vi "Process.vi"(8 "error in":errorcluster, 11 "JKI.Robot.SMO.TestUI":refnum<class "JKI.Robot.SMO.APITesterUI.lvclass">) -> (0 "error out":errorcluster, 3 "JKI.Robot.SMO.TestUI out":refnum<class "JKI.Robot.SMO.APITesterUI.lvclass">)   [LabVIEW 2015, in "JKI.Robot.SMO.APITesterUI.lvclass"]
doc: "---------------------------------------------------------------\nJKI State Machine Objects™\nhttp://jki.net/state-machine-objects/\nCopyright (C) 2005-2015, JKI <info@jki.net>\nALL RIGHTS RESERVEDJKI State Machine Objects (SMO) 1.0.0.5\nJKI - JKI\nCopyright (c) 2016, JKI"
uses:
  JKI.Robot.SMO.APITesterUI.lvclass
  <vilib>/JKI/JKI SMO/SMO/Typedefs/Parent Call--Enum.ctl
  JKI.Robot.SMO.APITesterUI.lvclass/JKI.Robot.SMO.APITesterUI.ctl
  JKI.Robot.SMO.Base/JKI.Robot.SMO.Base.lvclass
  <vilib>/JKI/JKI SMO/SMO.UI/SMO.UI.lvclass
  <vilib>/JKI/JKI SMO/SMO/SMO.lvclass
panel:
  in  "Joint C - Wrist":dbl(knob)=5.611498737356196 scale format="%#.1f"
  in  "Joint B - Elbow":dbl(knob)=5.611498737356196 scale format="%#.1f"
  in  "Joint A - Shoulder":dbl(knob)=5.611498737356196 scale format="%#.1f"
  in  "Claw Value":dbl(slide) scale=0.0..1.0
  # "For instructions on how to use the JKI State Machine Objects, examples and video tutorials, visit:\nhttp://jki.net/state-machine-objects/\n\nJKI State Machine Objects™\nhttp://jki.net/state-machine-objects/\nCopyright (C) 2005-2015, JKI <info@jki.net>\nALL RIGHTS RESERVED"
  # "LABVIEW CONTROLLER"
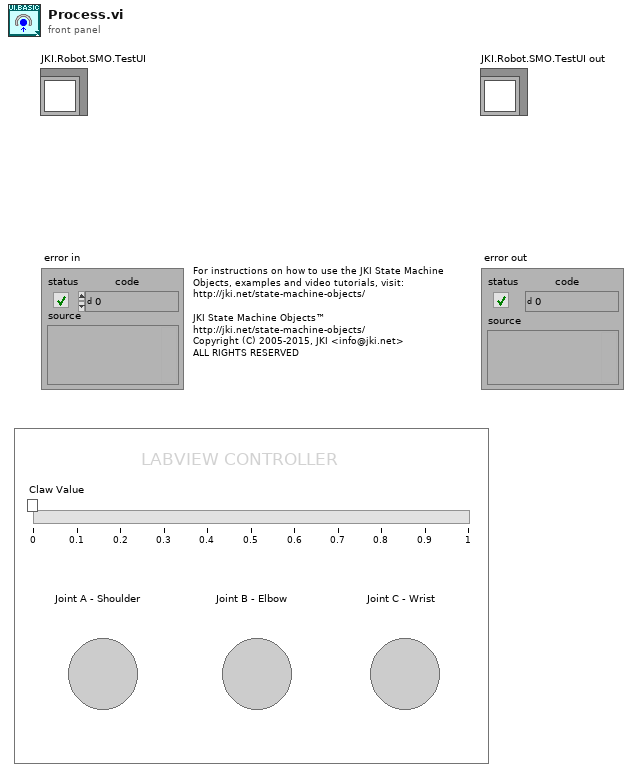
[diagram p1: front panel]
types:
  T1 = typedef "SMO.lvclass/Parent Call--Enum.ctl" = enum16{"Allows parent to run", "Does not request parent to run"}
  T2 = enum32{"invalid app kind", "Development System", "Run Time System", "Student Edition", "Embedded LabVIEW", "Evaluation", "Custom"}
  T3 = enum32{"Invalid", "Standard", "Closed", "Hidden", "Minimized", "Maximized"}
  T4 = cluster{"Core":cluster{"Current VI Reference":refnum<vi>, "Close Panel on Exit?":bool, "error":errorcluster}, "Self Reference":refnum<class "JKI.Robot.SMO.APITesterUI.lvclass">, "JKI.Robot":refnum<class "JKI.Robot.SMO.Base.lvclass">}
  T5 = cluster{"Current VI Reference":refnum<vi>, "Close Panel on Exit?":bool, "error":errorcluster}
  T6 = typedef "SMO.lvclass/Protected Events.ctl" = cluster{"StopProcesses":refnum<user-event>, "AbortProcesses":refnum<user-event>, "Config Changed":refnum<user-event>}
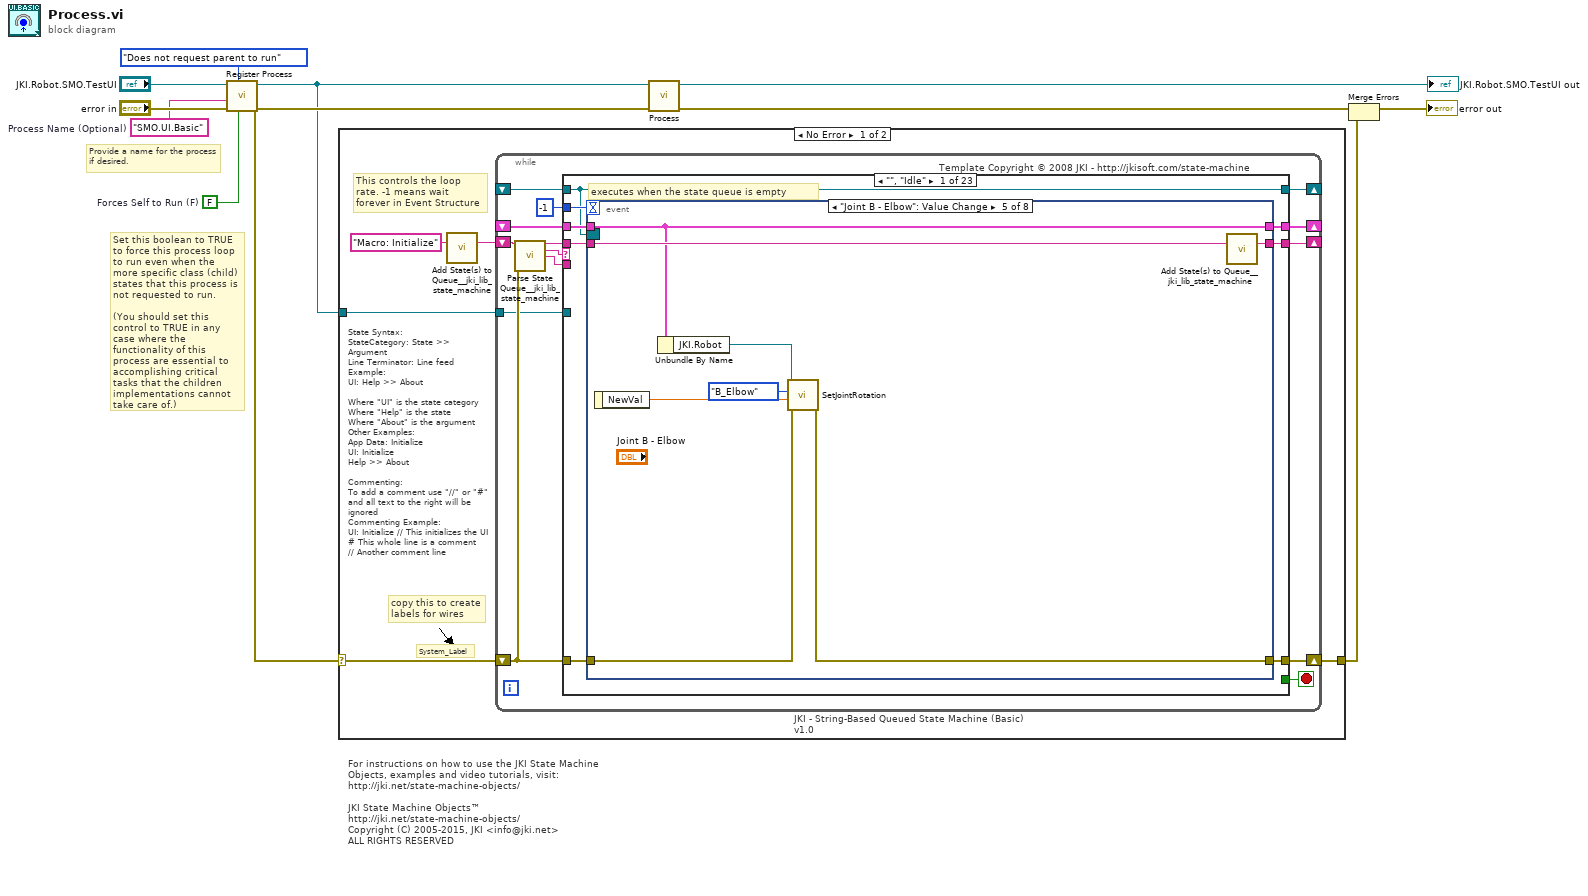
[diagram p0: block diagram]
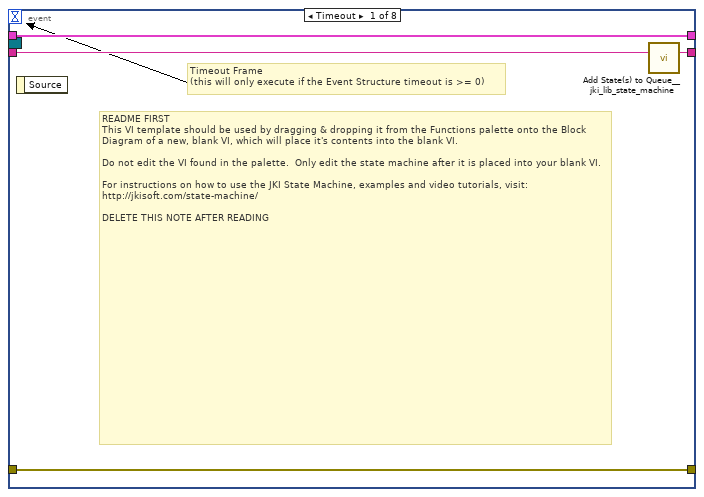
[diagram p2: hidden frame]
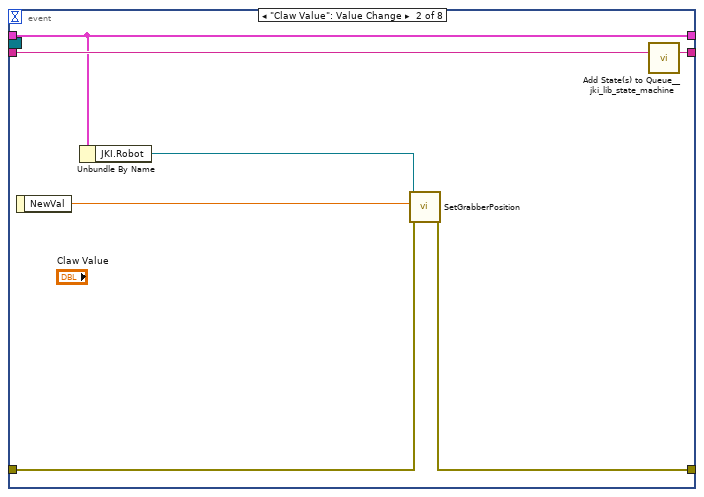
[diagram p3: hidden frame]
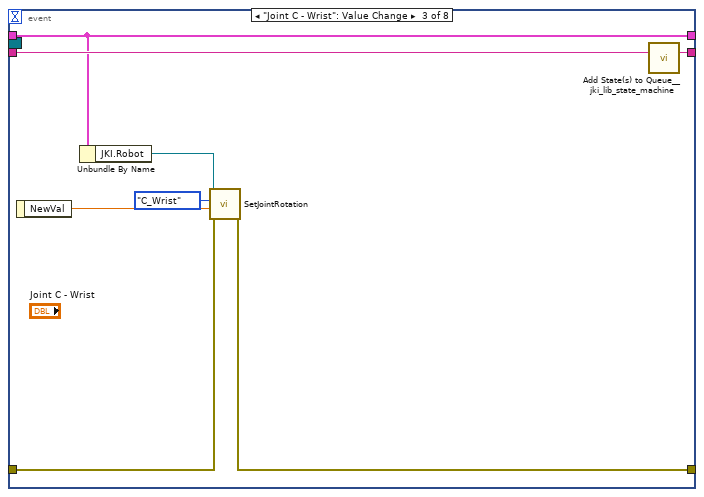
[diagram p4: hidden frame]
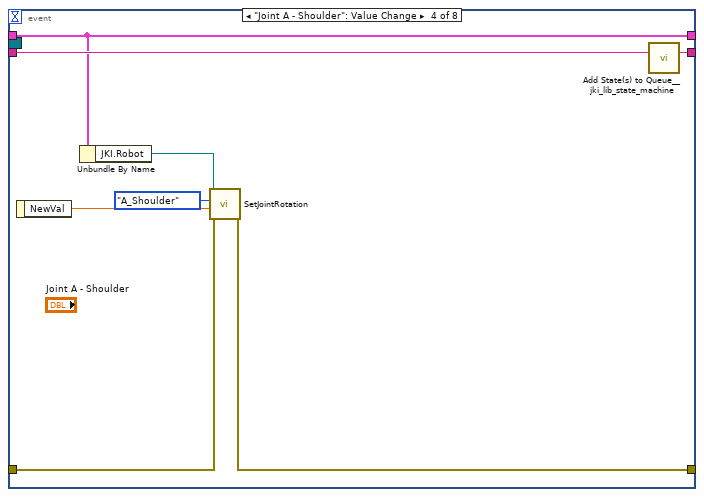
[diagram p5: hidden frame]
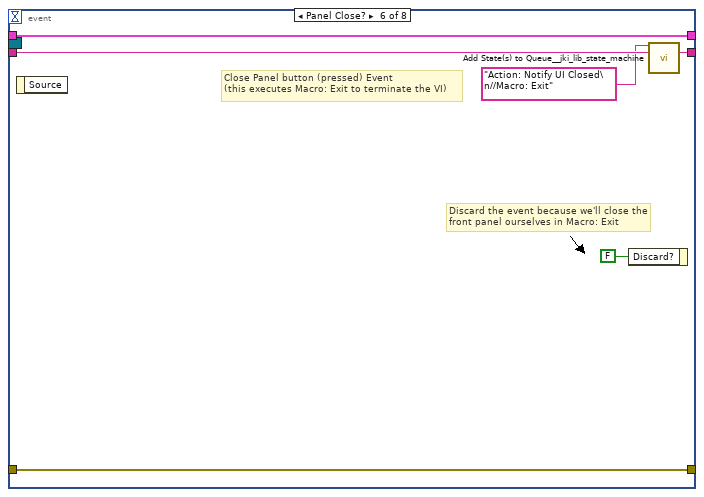
[diagram p6: hidden frame]
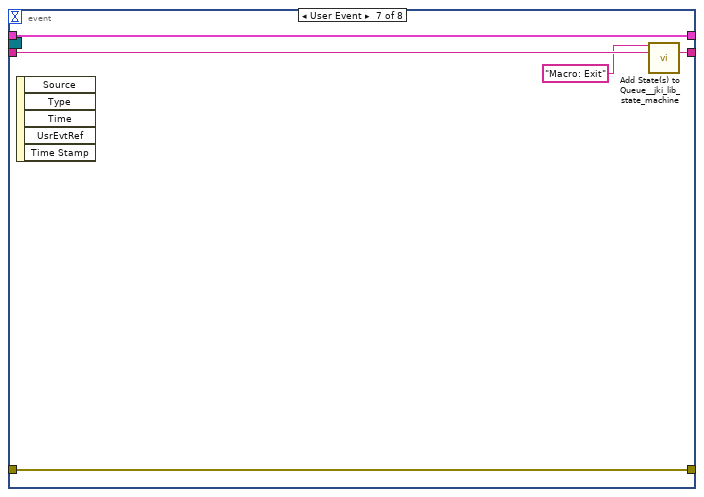
[diagram p7: hidden frame]
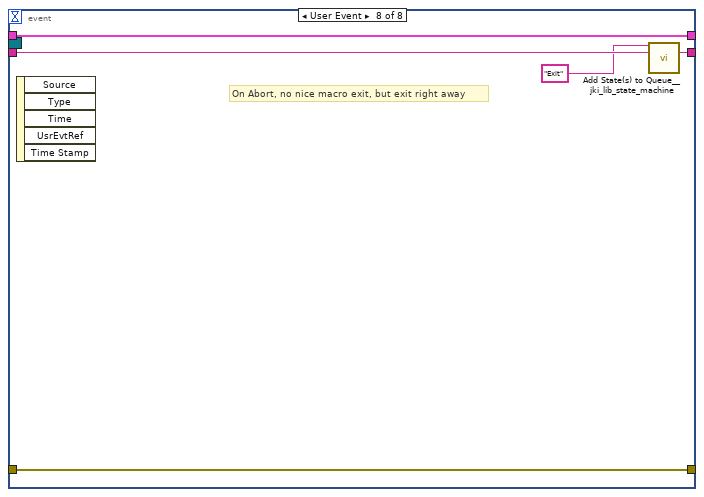
[diagram p8: hidden frame]
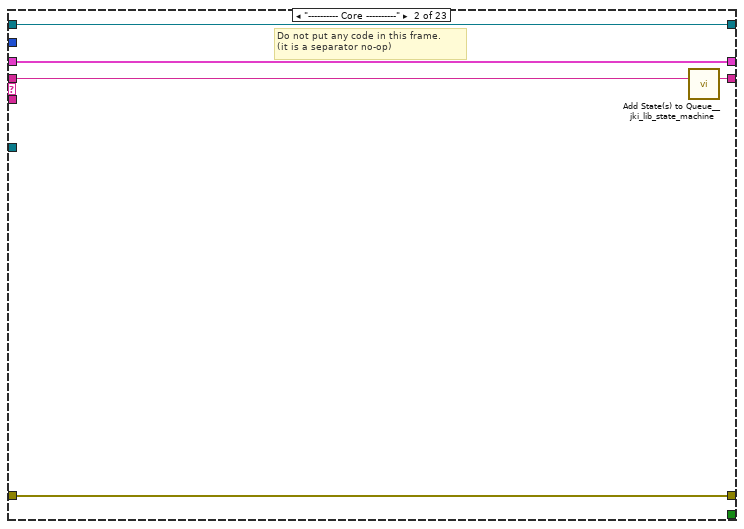
[diagram p9: hidden frame]
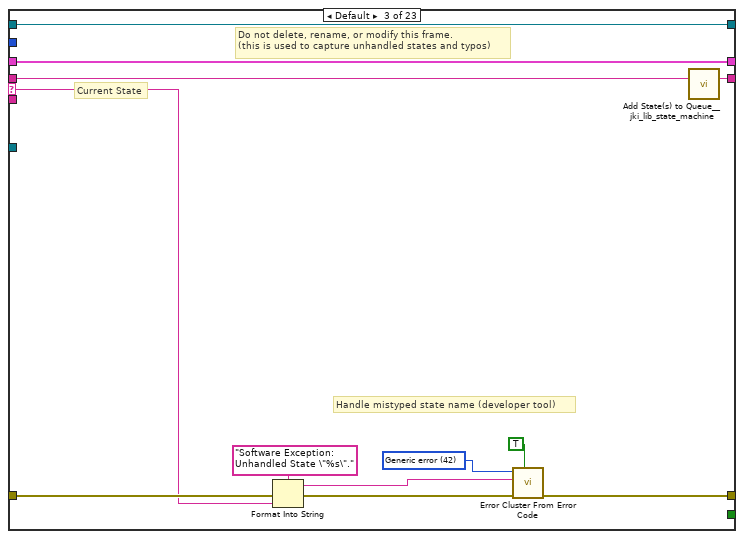
[diagram p10: hidden frame]
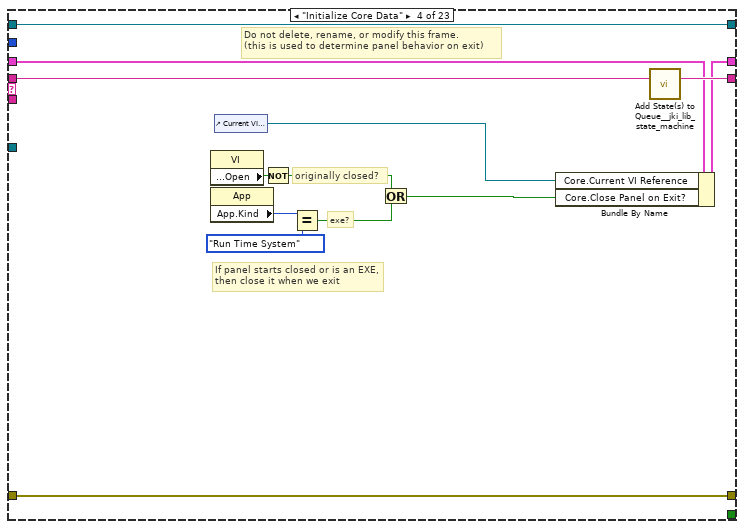
[diagram p11: hidden frame]
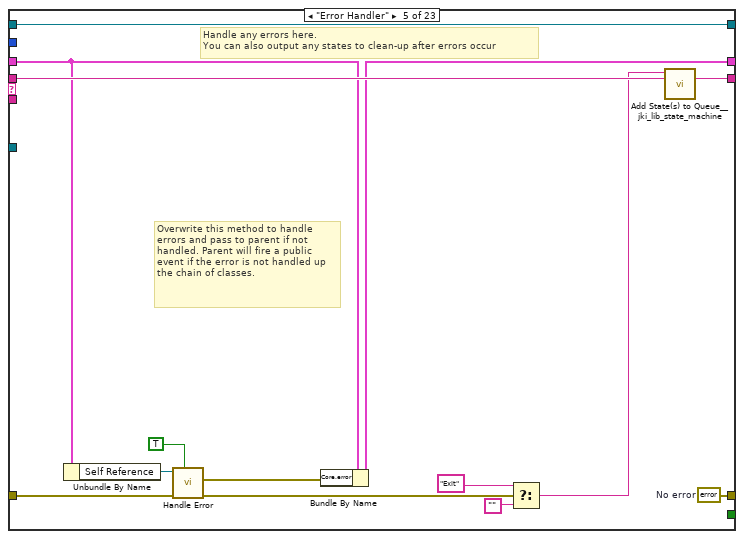
[diagram p12: hidden frame]
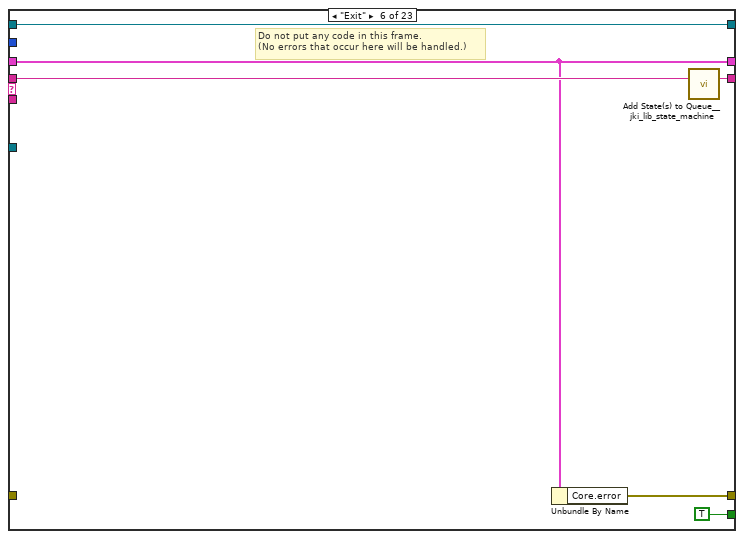
[diagram p13: hidden frame]
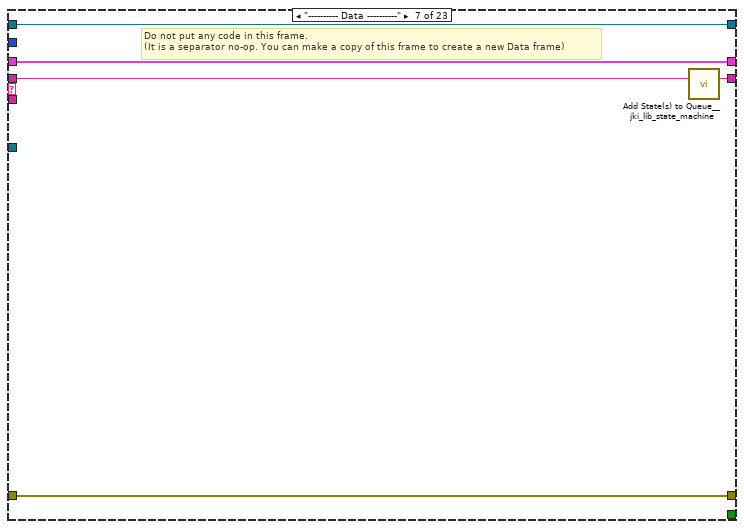
[diagram p14: hidden frame]
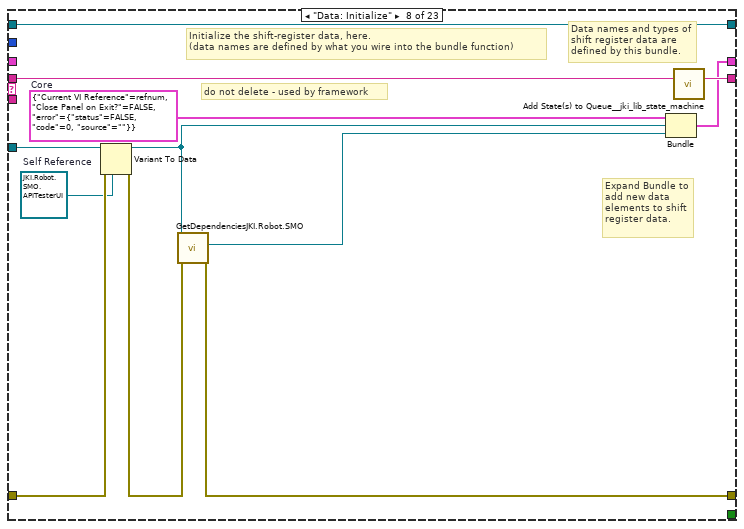
[diagram p15: hidden frame]
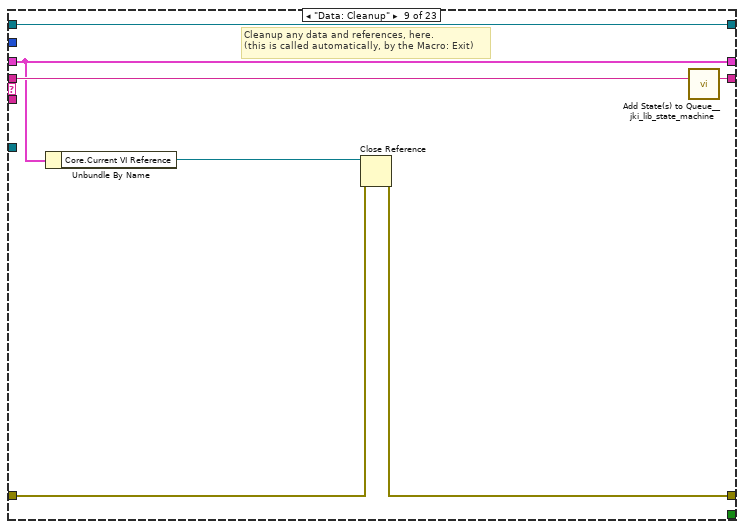
[diagram p16: hidden frame]
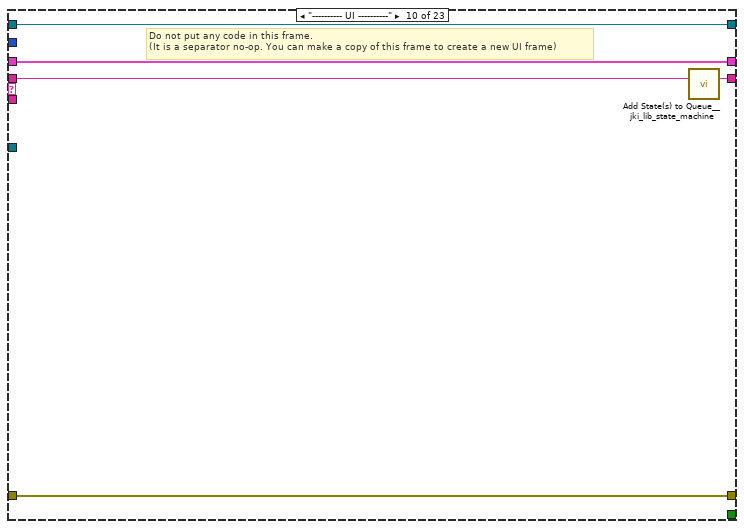
[diagram p17: hidden frame]
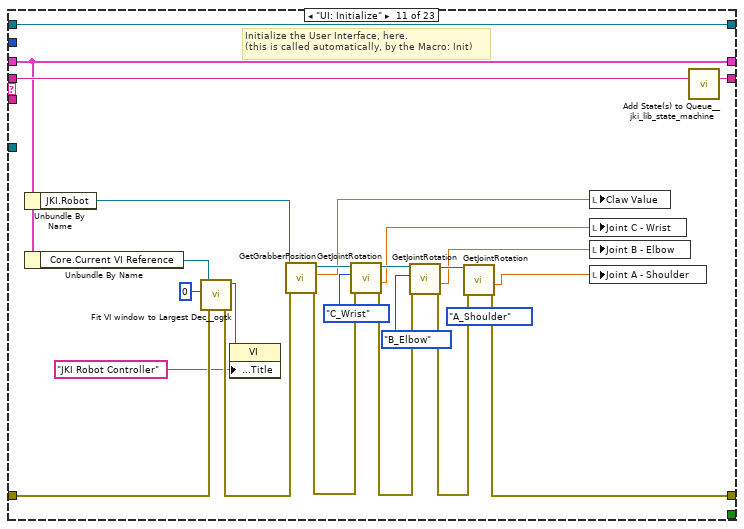
[diagram p18: hidden frame]
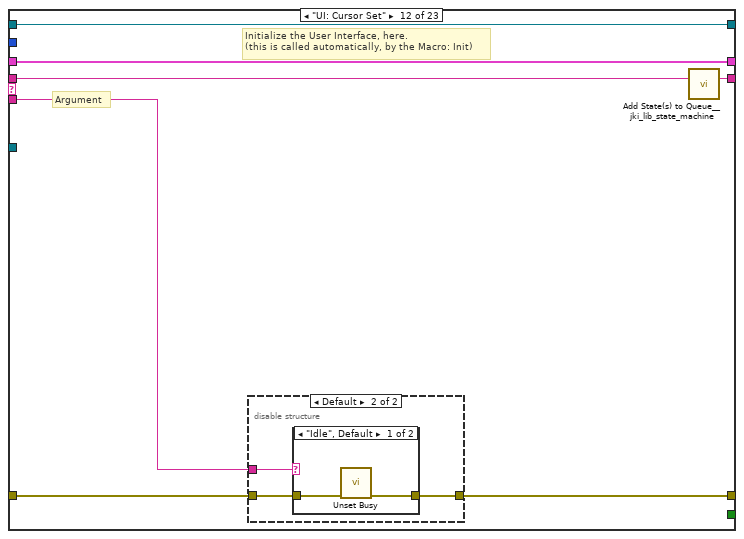
[diagram p19: hidden frame]
diagram:
  w2 = FALSE  # Forces Self to Run (F)
  w1 = "SMO.UI.Basic"  # Process Name (Optional)
  # "Provide a name for the process\nif desired."
  # "Set this boolean to TRUE to force this process loop to run even when the more specific class (child) states that this process is not requested to run.\n\n(You should set this control to TRUE in any case where the functionality of this process are essential to accomplishing critical tasks that the children implementations cannot take care of.)"
  # "For instructions on how to use the JKI State Machine Objects, examples and video tutorials, visit:\nhttp://jki.net/state-machine-objects/\n\nJKI State Machine Objects™\nhttp://jki.net/state-machine-objects/\nCopyright (C) 2005-2015, JKI <info@jki.net>\nALL RIGHTS RESERVED"
  n1 = call <vilib>:"Register Process.vi"("Forces Self to Run (F)"=w2, "Parent Call"=Parent_Call--Enum."Does not request parent to run", "error in (no error)"="error in", "Process Name (optional)"=w1, "SMO"="JKI.Robot.SMO.TestUI") -> ("error out"=w8:errorcluster, "SMO out"=w7:refnum<class "JKI.Robot.SMO.APITesterUI.lvclass">)  [unwired: 5 in]
  n2 = case shown="No Error" w8 {
    selector: w8 -> [w13 w333]
    tunnel: w7 -> [w14 _]
    tunnel: [w12 w333] -> w4
    frame No Error {
      # "State Syntax:\nStateCategory: State >> Argument\nLine Terminator: Line feed\nExample:\nUI: Help >> About\n\nWhere \"UI\" is the state category\nWhere \"Help\" is the state\nWhere \"About\" is the argument\nOther Examples:\nApp Data: Initialize\nUI: Initialize\nHelp >> About\n\nCommenting:\nTo add a comment use \"//\" or \"#\" and all text to the right will be ignored\nCommenting Example:\nUI: Initialize // This initializes the UI\n# This whole line is a comment\n// Another comment line"
      # "copy this to create labels for wires"
      # "This controls the loop rate. -1 means wait forever in Event Structure"
      # "System_Label"
      n3 = call <vilib>:"Add State(s) to Queue__jki_lib_state_machine.vi"("State(s) in (\"\")"="Macro: Initialize") -> ("States Out"=w16:string)  [unwired: 14 in]
      n4 = while "JKI - String-Based Queued State Machine (Basic) v1.0" {
        shift-right: [w23] -> _
        shift-left: _ -> [w22]
        shift-right: [w26] -> w12
        shift-left: w13 -> [w20]
        shift-right: [w25] -> _
        shift-left: w16 -> [w27]
        tunnel: w14 -> [w19]
        shift-right: [w18] -> _
        shift-left: _ -> [w17]
        stop <- w24 stop-if-true
        # "Template Copyright © 2008 JKI - http://jkisoft.com/state-machine"
        n5 = call <vilib>:"Parse State Queue__jki_lib_state_machine.vi"("State Queue"=w27, "Error In (no error)"=w20) -> ("Remaining States"=w29:string, "Current State"=w30:string, "Arguments"=w28:string)  [unwired: 11 in]
        n6 = case shown="\"\", \"Idle\"" w30 {
          selector: w30 -> [_ _ w96 _ _ _ _ _ _ _ _ _ _ _ _ _ _ _ _ _ _ _ _]
          tunnel: w29 -> [w38 w94 w100 w119 w133 w139 w144 w156 w163 w168 w193 w200 w216 w248 w257 w271 w276 w287 w292 w303 w318 w325 w332]
          tunnel: w28 -> [_ _ _ _ _ _ _ _ _ _ _ w194 w210 _ _ _ _ _ _ _ _ _ _]
          tunnel: w22 -> [w36 w91 w98 w110 w122 w135 w141 _ w158 w165 w174 w198 w212 w245 w253 w262 w273 w284 w289 w301 w316 w321 w328]
          tunnel: [w35 w92 w102 w116 w124 w134 w142 w146 w159 w166 w183 w195 w213 w246 w255 w269 w274 w278 w290 w299 w313 w322 w326] -> w26
          tunnel: w20 -> [w34 w92 w101 w116 w129 _ w142 w153 w160 w166 w172 w196 w214 w246 w255 w269 w274 w279 w290 w300 w314 w322 w327]
          tunnel: [w37 w93 w99 w118 w132 w138 w143 w155 w162 w167 w192 w199 w215 w247 w256 w270 w275 w286 w291 w302 w317 w324 w331] -> w25
          tunnel: [_ _ _ _ _ TRUE _ _ _ _ _ _ _ _ _ _ _ _ _ _ _ _ _] -> w24
          tunnel: [w33 w91 w98 w117 w121 w135 w141 w154 w158 w165 w174 w198 w212 w245 w253 w262 w273 w284 w289 w301 w316 w320 w328] -> w23
          tunnel: -1 ("Timeout") -> [w32 _ _ _ _ _ _ _ _ _ _ _ _ _ _ _ _ _ _ _ _ _ _]
          tunnel: w19 -> [_ _ _ _ _ _ _ w151 _ _ _ _ _ _ _ _ _ _ _ _ _ _ _]
          tunnel: [w31 w90 w95 w107 w131 w136 w140 w150 w157 w164 w191 w197 w209 w244 w254 w263 w272 w285 w288 w298 w315 w323 w330] -> w18
          tunnel: w17 -> [w31 w90 w95 w107 w131 w136 w140 w150 w157 w164 w191 w197 w209 w244 w254 w263 w272 w285 w288 w294 w315 w323 w330]
          frame "", "Idle" {
            # "executes when the state queue is empty"
            n7 = event shown="[4] \"Joint B - Elbow\": Value Change" {
              selector: w31 -> [_ _ _ _ _ _ _ _]
              dyn-events: _ -> [_ _ _ _ _ _ _ _]
              timeout: w32 -> [_ _ _ _ _ _ _ _]
              tunnel: w38 -> [w42 w49 w57 w65 w73 w79 w84 w89]
              tunnel: [w41 w48 w56 w64 w72 w78 w83 w88] -> w37
              tunnel: w36 -> [w39 w47 w55 w63 w71 w75 w81 w86]
              tunnel: [w40 w43 w52 w60 w68 w74 w82 w87] -> w35
              tunnel: w34 -> [w40 w44 w53 w61 w69 w74 w82 w87]
              tunnel: [w39 w47 w55 w63 w71 w75 w81 w86] -> w33
              event Timeout {
                # "README FIRST\nThis VI template should be used by dragging & dropping it from the Functions palette onto the Block Diagram of a new, blank VI, which will place it's contents into the blank VI.\n\nDo not edit the VI found in the palette.  Only edit the state machine after it is placed into your blank VI.\n\nFor instructions on how to use the JKI State Machine, examples and video tutorials, visit:\nhttp://jkisoft.com/state-machine/\n\nDELETE THIS NOTE AFTER READING"
                # "Timeout Frame\n(this will only execute if the Event Structure timeout is >= 0)"
                n8 = event-data() -> ()  [unwired: 1 in, 1 out]
                n9 = call <vilib>:"Add State(s) to Queue__jki_lib_state_machine.vi"("State(s) in (\"\")"=w42) -> ("States Out"=w41:string)  [unwired: 14 in]
              }
              event "Claw Value": Value Change {
                n10 = event-data() -> ("NewVal"=w45:dbl)  [unwired: 1 in]
                n11 = Unbundle By Name(w47) -> ("JKI.Robot"=w46:refnum<class "JKI.Robot.SMO.Base.lvclass">)
                n12 = call-dynamic "SetGrabberPosition.vi"("error in (no error)"=w44, "GrabberPosition"=w45, "JKI.Robot"=w46) -> ("error out"=w43:errorcluster)  [unwired: 7 in, 1 out]
                n13 = call <vilib>:"Add State(s) to Queue__jki_lib_state_machine.vi"("State(s) in (\"\")"=w49) -> ("States Out"=w48:string)  [unwired: 14 in]
              }
              event "Joint C - Wrist": Value Change {
                n14 = event-data() -> ("NewVal"=w51:dbl)  [unwired: 1 in]
                n15 = Unbundle By Name(w55) -> ("JKI.Robot"=w54:refnum<class "JKI.Robot.SMO.Base.lvclass">)
                n16 = call-dynamic "SetJointRotation.vi"("error in (no error)"=w53, "Rotation (Deg)"=w51, "Joint"=enum16{"A_Shoulder", "B_Elbow", "C_Wrist"}."C_Wrist" ("JointType"), "JKI.Robot.SMO.Base"=w54) -> ("error out"=w52:errorcluster)  [unwired: 6 in, 1 out]
                n17 = call <vilib>:"Add State(s) to Queue__jki_lib_state_machine.vi"("State(s) in (\"\")"=w57) -> ("States Out"=w56:string)  [unwired: 14 in]
              }
              event "Joint A - Shoulder": Value Change {
                n18 = event-data() -> ("NewVal"=w59:dbl)  [unwired: 1 in]
                n19 = Unbundle By Name(w63) -> ("JKI.Robot"=w62:refnum<class "JKI.Robot.SMO.Base.lvclass">)
                n20 = call-dynamic "SetJointRotation.vi"("error in (no error)"=w61, "Rotation (Deg)"=w59, "Joint"=enum16{"A_Shoulder", "B_Elbow", "C_Wrist"}."A_Shoulder" ("JointType"), "JKI.Robot.SMO.Base"=w62) -> ("error out"=w60:errorcluster)  [unwired: 6 in, 1 out]
                n21 = call <vilib>:"Add State(s) to Queue__jki_lib_state_machine.vi"("State(s) in (\"\")"=w65) -> ("States Out"=w64:string)  [unwired: 14 in]
              }
              event "Joint B - Elbow": Value Change {
                n22 = event-data() -> ("NewVal"=w67:dbl)  [unwired: 1 in]
                n23 = Unbundle By Name(w71) -> ("JKI.Robot"=w70:refnum<class "JKI.Robot.SMO.Base.lvclass">)
                n24 = call-dynamic "SetJointRotation.vi"("error in (no error)"=w69, "Rotation (Deg)"=w67, "Joint"=enum16{"A_Shoulder", "B_Elbow", "C_Wrist"}."B_Elbow" ("JointType"), "JKI.Robot.SMO.Base"=w70) -> ("error out"=w68:errorcluster)  [unwired: 6 in, 1 out]
                n25 = call <vilib>:"Add State(s) to Queue__jki_lib_state_machine.vi"("State(s) in (\"\")"=w73) -> ("States Out"=w72:string)  [unwired: 14 in]
              }
              event Panel Close? {
                # "Discard the event because we'll close the front panel ourselves in Macro: Exit"
                # "Close Panel button (pressed) Event\n(this executes Macro: Exit to terminate the VI)"
                n26 = event-data() -> ()  [unwired: 1 in, 1 out]
                n27 = event-data("Discard?"=FALSE) -> ()  [unwired: 1 in, 1 out]
                n28 = call <vilib>:"Add State(s) to Queue__jki_lib_state_machine.vi"("State(s) in Front (\"\")"="Action: Notify UI Closed\n//Macro: Exit", "State(s) in (\"\")"=w79) -> ("States Out"=w78:string)  [unwired: 13 in]
              }
              event User Event {
                n29 = event-data() -> ()  [unwired: 1 in, 5 out]
                n30 = call <vilib>:"Add State(s) to Queue__jki_lib_state_machine.vi"("State(s) in Front (\"\")"="Macro: Exit", "State(s) in (\"\")"=w84) -> ("States Out"=w83:string)  [unwired: 13 in]
              }
              event User Event {
                # "On Abort, no nice macro exit, but exit right away"
                n31 = event-data() -> ()  [unwired: 1 in, 5 out]
                n32 = call <vilib>:"Add State(s) to Queue__jki_lib_state_machine.vi"("State(s) in Front (\"\")"="Exit", "State(s) in (\"\")"=w89) -> ("States Out"=w88:string)  [unwired: 13 in]
              }
            }
          }
          frame "---------- Core ----------" {
            # "Do not put any code in this frame.\n(it is a separator no-op)"
            n33 = call <vilib>:"Add State(s) to Queue__jki_lib_state_machine.vi"("State(s) in (\"\")"=w94) -> ("States Out"=w93:string)  [unwired: 14 in]
          }
          frame Default {
            w105 = 42 items=["No error", "Argument error", "Memory is full", "Out of zone", "End of file", "File already open", "Generic file I/O error", "File not found", "File permission error", "Disk is full", "Duplicate path", "Too many files open", "System feature not enabled", "Resource file not found", "Cannot add resource", "Resource not found", "Image not found", "Image memory error", "Pen does not exist", "Config type invalid", "Config token not found", "Config parse error", "Config memory error", "Bad external code format", "Bad external code offset", "External code not present", "Null window", "Destroy window error", "Null menu", "Print aborted", "Bad print record", "Print driver error", "Windows error during printing", "Memory error during printing", "Print dialog error", "Generic print error", "Invalid device refnum", "Device not found", "Device parameter error", "Device unit error", "Cannot open device", "Device call aborted", "Generic error", "Cancelled by user", "Object ID too low", "Object ID too high", "Object not in heap", "Unknown heap", "Unknown object (invalid DefProc)", "Unknown object (DefProc not in table)", "Message out of range", "Invalid (null) method", "Unknown message", "Manager call not supported", "Bad address", "Network operation in progress", "Network operation timed out", "Connection is busy", "Network attribute not supported", "Network error", "Address in use", "System out of memory", "Connection aborted", "Connection refused", "Not connected", "Already connected", "Connection closed", "Initialization error (interapplication manager)", "Bad occurrence", "Wait on unbound occurrence handler", "Occurrence queue overflow", "Datalog type conflict", "Unused", "Unrecognized type (interapplication manager)", "Memory corrupt", "Failed to make temporary DLL", "Old CIN version", "Drag socket not found", "Failed to load drop-object", "Failed to register OLE object", "Failed to release OLE object", "Format specifier type mismatch", "Unknown format specifier", "Too few format specifiers", "Too many format specifiers", "Scan failed", "Newer CIN version", "Error converting to variant", "Runtime menu error", "Password tampered", "Variant attribute not found", "Incompatible variant data type", "Event data is not available", "Event Store is not present", "Occurrence is not found", "Event Queue is not created", "Event info is not available", "Refnum passed is NULL", "Error retrieving Class GUID", "Error retrieving CoClass GUID", "Error retrieving TypeLib GUID.", "Bad built application magic bytes.", "Specific driver is different from the specific driver associated with the Logical Name.", "There is no session opened to the class driver.", "Max Error", "MAX - Error with config objects", "MAX - Error loading configuration", "MAX - Group not supported"]
            # "Current State"
            # "Do not delete, rename, or modify this frame.\n(this is used to capture unhandled states and typos)"
            # "Handle mistyped state name (developer tool)"
            n34 = Format Into String(format string="Software Exception: Unhandled State \"%s\"." ("message"), error in=w101, w96) -> (resulting string=w104:string, error out=w103:errorcluster)  [unwired: 1 in]
            n35 = call <vilib>:"Error Cluster From Error Code.vi"("show call chain? (False)"=TRUE, "error in (no error)"=w103, "error message (\"\")"=w104, "error code (0)"=w105) -> ("error out"=w102:errorcluster)  [unwired: 5 in]
            n36 = call <vilib>:"Add State(s) to Queue__jki_lib_state_machine.vi"("State(s) in (\"\")"=w100) -> ("States Out"=w99:string)  [unwired: 14 in]
          }
          frame "Initialize Core Data" {
            # "Do not delete, rename, or modify this frame.\n(this is used to determine panel behavior on exit)"
            # "originally closed?"
            # "exe?"
            # "If panel starts closed or is an EXE, then close it when we exit"
            n37 = property class="VI"() -> ("Front Panel.Open"=w115:bool)  [unwired: 2 in, 2 out]
            n38 = property class="App"() -> ("App.Kind"=w114:T2)  [unwired: 2 in, 2 out]
            n39 = control-ref of="Current VI Reference"() -> (w108:refnum<vi>)
            n40 = Not(x=w115) -> (.not. x?=w112:bool)
            n41 = Equal?(x=w114, y=T2."Run Time System" ("Application:Kind")) -> (x = y?=w111:bool)
            n42 = Or(x=w112, y=w111) -> (x .or. y?=w109:bool)
            n43 = Bundle By Name(cluster=w110, "Core.Current VI Reference"=w108, "Core.Close Panel on Exit?"=w109) -> (w117:T4)
            n44 = call <vilib>:"Add State(s) to Queue__jki_lib_state_machine.vi"("State(s) in (\"\")"=w119) -> ("States Out"=w118:string)  [unwired: 14 in]
          }
          frame "Error Handler" {
            w124 = errorcluster {"status"=FALSE, "code"=0, "source"=""}  # No error
            # "Overwrite this method to handle errors and pass to parent if not handled. Parent will fire a public event if the error is not handled up the chain of classes."
            # "Handle any errors here.\nYou can also output any states to clean-up after errors occur"
            n45 = Unbundle By Name(w122) -> ("Self Reference"=w130:refnum<class "JKI.Robot.SMO.APITesterUI.lvclass">)
            n46 = call-dynamic "Handle Error.vi"("Stop on Unhandled Error (T)"=TRUE, "error in"=w129, "SMO"=w130) -> ("handling error"=w125:errorcluster, "Unhandled error"=w123:errorcluster)  [unwired: 6 in, 1 out]
            n47 = Bundle By Name(cluster=w122, "Core.error"=w123) -> (w121:T4)
            n48 = Select(t="Exit", s=w125, f="") -> (s? t:f=w126:string)
            n49 = call <vilib>:"Add State(s) to Queue__jki_lib_state_machine.vi"("State(s) in Front (\"\")"=w126, "State(s) in (\"\")"=w133) -> ("States Out"=w132:string)  [unwired: 13 in]
          }
          frame "Exit" {
            # "Do not put any code in this frame.\n(No errors that occur here will be handled.)"
            n50 = Unbundle By Name(w135) -> ("Core.error"=w134:errorcluster)
            n51 = call <vilib>:"Add State(s) to Queue__jki_lib_state_machine.vi"("State(s) in (\"\")"=w139) -> ("States Out"=w138:string)  [unwired: 14 in]
          }
          frame "---------- Data ----------" {
            # "Do not put any code in this frame.\n(It is a separator no-op. You can make a copy of this frame to create a new Data frame)"
            n52 = call <vilib>:"Add State(s) to Queue__jki_lib_state_machine.vi"("State(s) in (\"\")"=w144) -> ("States Out"=w143:string)  [unwired: 14 in]
          }
          frame "Data: Initialize" {
            w149 = T5 {"Current VI Reference"=refnum, "Close Panel on Exit?"=FALSE, "error"={"status"=FALSE, "code"=0, "source"=""}}  # Core
            w152 = refnum<class "JKI.Robot.SMO.APITesterUI.lvclass"> refnum  # Self Reference
            # "do not delete - used by framework"
            # "Expand Bundle to add new data elements to shift register data."
            # "Data names and types of shift register data are defined by this bundle."
            # "Initialize the shift-register data, here.\n(data names are defined by what you wire into the bundle function)"
            n53 = Variant To Data(error in=w153, type=w152, Variant=w151) -> (data=w148:refnum<class "JKI.Robot.SMO.APITesterUI.lvclass">, error out=w147:errorcluster)
            n54 = call "GetDependenciesJKI.Robot.SMO.vi"("error in (no error)"=w147, "JKI.Robot.SMO.APITesterUI in"=w148) -> ("error out"=w146:errorcluster, "JKI.Robot"=w145:refnum<class "JKI.Robot.SMO.Base.lvclass">)  [unwired: 7 in, 1 out]
            n55 = Bundle("Core"=w149, "Self Reference"=w148, "JKI.Robot"=w145) -> (w154:T4)  [unwired: 1 in]
            n56 = call <vilib>:"Add State(s) to Queue__jki_lib_state_machine.vi"("State(s) in (\"\")"=w156) -> ("States Out"=w155:string)  [unwired: 14 in]
          }
          frame "Data: Cleanup" {
            # "Cleanup any data and references, here.\n(this is called automatically, by the Macro: Exit)"
            n57 = Unbundle By Name(w158) -> ("Core.Current VI Reference"=w161:refnum<vi>)
            n58 = Close Reference(reference=w161, error in (no error)=w160) -> (error out=w159:errorcluster)
            n59 = call <vilib>:"Add State(s) to Queue__jki_lib_state_machine.vi"("State(s) in (\"\")"=w163) -> ("States Out"=w162:string)  [unwired: 14 in]
          }
          frame "---------- UI ----------" {
            # "Do not put any code in this frame.\n(It is a separator no-op. You can make a copy of this frame to create a new UI frame)"
            n60 = call <vilib>:"Add State(s) to Queue__jki_lib_state_machine.vi"("State(s) in (\"\")"=w168) -> ("States Out"=w167:string)  [unwired: 14 in]
          }
          frame "UI: Initialize" {
            # "Initialize the User Interface, here.\n(this is called automatically, by the Macro: Init)"
            n61 = Unbundle By Name(w174) -> ("JKI.Robot"=w190:refnum<class "JKI.Robot.SMO.Base.lvclass">)
            n62 = Unbundle By Name(w174) -> ("Core.Current VI Reference"=w173:refnum<vi>)
            n63 = call <userlib>:"Fit VI window to Largest Dec__ogtk.vi"("error in (no error)"=w172, "border spacing (2 px)"=0, "VI Ref (calling VI)"=w173) -> ("error out"=w171:errorcluster, "dup VI Ref"=w170:refnum<vi>)  [unwired: 3 in]
            n64 = property class="VI"(reference=w170, "Front Panel.Title"="JKI Robot Controller" ("Front Panel Window:Title")) -> ()  [unwired: 1 in, 2 out]
            n65 = call-dynamic "GetGrabberPosition.vi"("error in (no error)"=w171, "JKI.Robot.SMO.Base.lvclass"=w190) -> ("error out"=w186:errorcluster, "SetGrabberPosition"=w182:dbl, "JKI.Robot.SMO.Base.lvclass"=w189:refnum<class "JKI.Robot.SMO.Base.lvclass">)  [unwired: 7 in]
            n66 = call-dynamic "GetJointRotation.vi"("error in (no error)"=w186, "Joint"=enum16{"A_Shoulder", "B_Elbow", "C_Wrist"}."C_Wrist" ("JointType"), "JKI.Robot.SMO.Base"=w189) -> ("error out"=w185:errorcluster, "Rotation (Deg)"=w181:dbl, "JKI.Robot.SMO.Base"=w188:refnum<class "JKI.Robot.SMO.Base.lvclass">)  [unwired: 6 in]
            n67 = call-dynamic "GetJointRotation.vi"("error in (no error)"=w185, "Joint"=enum16{"A_Shoulder", "B_Elbow", "C_Wrist"}."B_Elbow" ("JointType"), "JKI.Robot.SMO.Base"=w188) -> ("error out"=w184:errorcluster, "Rotation (Deg)"=w180:dbl, "JKI.Robot.SMO.Base"=w187:refnum<class "JKI.Robot.SMO.Base.lvclass">)  [unwired: 6 in]
            n68 = call-dynamic "GetJointRotation.vi"("error in (no error)"=w184, "Joint"=enum16{"A_Shoulder", "B_Elbow", "C_Wrist"}."A_Shoulder" ("JointType"), "JKI.Robot.SMO.Base"=w187) -> ("error out"=w183:errorcluster, "Rotation (Deg)"=w179:dbl)  [unwired: 6 in, 1 out]
            n69 = local write "Claw Value"(w182) -> ()
            n70 = local write "Joint C - Wrist"(w181) -> ()
            n71 = local write "Joint B - Elbow"(w180) -> ()
            n72 = local write "Joint A - Shoulder"(w179) -> ()
            n73 = call <vilib>:"Add State(s) to Queue__jki_lib_state_machine.vi"("State(s) in (\"\")"=w193) -> ("States Out"=w192:string)  [unwired: 14 in]
          }
          frame "UI: Cursor Set" {
            # "Argument"
            # "Initialize the User Interface, here.\n(this is called automatically, by the Macro: Init)"
            n74 = disable-structure shown="Default" {
              disable-tunnel: w196 -> [w201 w204]
              disable-tunnel: [w201 w203] -> w195
              disable-tunnel: w194 -> [_ w202]
              frame condition #0 {
              }
              frame condition #1 (active) {
                n75 = case shown="\"Idle\", Default" w202 {
                  tunnel: w204 -> [w206 w208]
                  tunnel: [w205 w207] -> w203
                  frame "Idle", Default {
                    n76 = call <vilib>:"Unset Busy.vi"("error in (no error)"=w206) -> ("error out"=w205:errorcluster)  [unwired: 10 in]
                  }
                  frame "Busy" {
                    n77 = call <vilib>:"Set Busy.vi"("error in (no error)"=w208) -> ("error out"=w207:errorcluster)  [unwired: 9 in, 1 out]
                  }
                }
              }
            }
            n78 = call <vilib>:"Add State(s) to Queue__jki_lib_state_machine.vi"("State(s) in (\"\")"=w200) -> ("States Out"=w199:string)  [unwired: 14 in]
          }
          frame "UI: Front Panel State" {
            # "Argument"
            # "Set Front Panel Open or Closed\n(Usage: \"UI: Front Panel State >> Open|Close\")"
            n79 = Unbundle By Name(w212) -> ("Core.Current VI Reference"=w211:refnum<vi>)
            n80 = disable-structure shown="Default" {
              disable-tunnel: w214 -> [w220 w243]
              disable-tunnel: [w219 w243] -> w213
              disable-tunnel: w211 -> [w218 _]
              disable-tunnel: w210 -> [w217 _]
              frame condition #0 (active) {
                n81 = case shown="\"Close\"" w217 {
                  tunnel: w220 -> [w224 w237]
                  tunnel: [w226 w238] -> w219
                  tunnel: w218 -> [w225 w235]
                  frame "Open", Default {
                    n82 = property class="VI"(reference=w225, error in=w224) -> (reference out=w222:refnum<vi>, error out=w223:errorcluster, "FP.State"=w221:T3)
                    n83 = case shown="\"Closed\"" w221 {
                      tunnel: [w229 w232] -> w226
                      tunnel: w223 -> [w228 w232]
                      tunnel: w222 -> [w227 _]
                      frame "Closed" {
                        n84 = invoke class="VI" method="FP.Open"(reference=w227, error in=w228, "Activate"=TRUE, "State"=T3."Standard") -> (error out=w229:errorcluster)  [unwired: 1 in, 4 out]
                      }
                      frame Default {
                      }
                    }
                  }
                  frame "Close" {
                    n85 = property class="VI"(reference=w235, error in=w237) -> (reference out=w234:refnum<vi>, error out=w236:errorcluster, "FP.State"=w233:T3)
                    n86 = case shown="Default" w233 {
                      tunnel: [w239 w242] -> w238
                      tunnel: w236 -> [w239 w241]
                      tunnel: w234 -> [_ w240]
                      frame "Invalid", "Closed" {
                      }
                      frame Default {
                        n87 = invoke class="VI" method="FP.Close"(reference=w240, error in=w241) -> (error out=w242:errorcluster)  [unwired: 1 in, 2 out]
                      }
                    }
                  }
                }
              }
              frame condition #1 {
              }
            }
            n88 = call <vilib>:"Add State(s) to Queue__jki_lib_state_machine.vi"("State(s) in (\"\")"=w216) -> ("States Out"=w215:string)  [unwired: 14 in]
          }
          frame "---------- Macro ----------" {
            # "Do not put any code in this frame.\n(It is a separator no-op. You can make a copy of this frame to create a new Macro frame)"
            n89 = call <vilib>:"Add State(s) to Queue__jki_lib_state_machine.vi"("State(s) in (\"\")"=w248) -> ("States Out"=w247:string)  [unwired: 14 in]
          }
          frame "Macro: Initialize" {
            w251 = "UI: Initialize\n//UI: Front Panel State >> Open"  # UI: Initialize //UI: Front Panel State >> Open
            # "Initialization Macro\n(This is called once, when the VI starts)"
            n90 = call <vilib>:"Add State(s) to Queue__jki_lib_state_machine.vi"("State(s) in Front (\"\")"="Data: Initialize\nInitialize Core Data\nEvents: Register", "State(s) in (\"\")"="Process: Sync", "State(s) at Back (\"\")"=w251) -> ("States Out"=w250:string)  [unwired: 12 in]
            n91 = call <vilib>:"Add State(s) to Queue__jki_lib_state_machine.vi"("State(s) in Front (\"\")"=w250, "State(s) in (\"\")"=w257) -> ("States Out"=w256:string)  [unwired: 13 in]
          }
          frame "Macro: Exit" {
            # "Exit Macro\n(This is called once, when the VI exits)"
            n92 = Unbundle By Name(w262) -> ("Core.Close Panel on Exit?"=w268:bool)
            n93 = Select(t="//UI: Front Panel State >> Close", s=w268, f="") -> (s? t:f=w265:string)
            n94 = call <vilib>:"Add State(s) to Queue__jki_lib_state_machine.vi"("State(s) in Front (\"\")"="Data: Cleanup\nEvents: Unregister", "State(s) in (\"\")"="Process: Sync", "State(s) at Back (\"\")"="Exit") -> ("States Out"=w259:string)  [unwired: 12 in]
            n95 = call <vilib>:"Add State(s) to Queue__jki_lib_state_machine.vi"("State(s) in (\"\")"=w265, "State(s) at Back (\"\")"=w259) -> ("States Out"=w264:string)  [unwired: 13 in]
            n96 = call <vilib>:"Add State(s) to Queue__jki_lib_state_machine.vi"("State(s) in Front (\"\")"=w264, "State(s) in (\"\")"=w271) -> ("States Out"=w270:string)  [unwired: 13 in]
          }
          frame "---------- Process ----------" {
            # "Template Separator\n(You can make a copy of, or modify, this frame)"
            n97 = call <vilib>:"Add State(s) to Queue__jki_lib_state_machine.vi"("State(s) in (\"\")"=w276) -> ("States Out"=w275:string)  [unwired: 14 in]
          }
          frame "Process: Sync" {
            n98 = Unbundle By Name(w284) -> ("Self Reference"=w280:refnum<class "JKI.Robot.SMO.APITesterUI.lvclass">)
            n99 = call <vilib>:"WaitOnProcessSync.vi"("error in (no error)"=w279, "SMO"=w280) -> ("error out"=w278:errorcluster, "Don't run?"=w283:bool)  [unwired: 7 in, 1 out]
            n100 = Select(t="Data: Cleanup\nEvents: Unregister\nExit", s=w283, f="") -> (s? t:f=w277:string)
            n101 = call <vilib>:"Add State(s) to Queue__jki_lib_state_machine.vi"("State(s) in Front (\"\")"=w277, "State(s) in (\"\")"=w287) -> ("States Out"=w286:string)  [unwired: 13 in]
          }
          frame "---------- Events ----------" {
            # "Template Separator\n(You can make a copy of, or modify, this frame)"
            n102 = call <vilib>:"Add State(s) to Queue__jki_lib_state_machine.vi"("State(s) in (\"\")"=w292) -> ("States Out"=w291:string)  [unwired: 14 in]
          }
          frame "Events: Register" {
            # "Self Events (API Calls)"
            # "Base Class Protected Events"
            n103 = Unbundle By Name(w301) -> ("Self Reference"=w296:refnum<class "JKI.Robot.SMO.APITesterUI.lvclass">)
            n104 = call <vilib>:"GetProtectedEvents.vi"("error in (no error)"=w300, "SMO"=w296) -> ("error out"=w293:errorcluster, "SMO Protected Events"=w297:T6)  [unwired: 7 in, 1 out]
            n105 = Not A Number/Path/Refnum?(number/path/refnum=w294) -> (NaN/Path/Refnum?=w295:bool)
            n106 = case shown="False" w295 {
              tunnel: [w307 w312] -> w299
              tunnel: [w306 w311] -> w298
              tunnel: w297 -> [w305 w310]
              tunnel: w293 -> [w304 w309]
              tunnel: w294 -> [_ w308]
              frame True {
                # "Expand to add\nmore events"
                n107 = register-events(error in=w304, w305) -> (reference out=w306:refnum<event-registration>, error out=w307:errorcluster)  [unwired: 1 in]
              }
              frame False {
                n108 = register-events(reference=w308, error in=w309, w310) -> (reference out=w311:refnum<event-registration>, error out=w312:errorcluster)
              }
            }
            n109 = call <vilib>:"Add State(s) to Queue__jki_lib_state_machine.vi"("State(s) in (\"\")"=w303) -> ("States Out"=w302:string)  [unwired: 14 in]
          }
          frame "Events: Unregister" {
            n110 = Unregister For Events(event registration refnum=w315, error in=w314) -> (error out=w313:errorcluster)
            n111 = call <vilib>:"Add State(s) to Queue__jki_lib_state_machine.vi"("State(s) in (\"\")"=w318) -> ("States Out"=w317:string)  [unwired: 14 in]
          }
          frame "---------- Action ----------" {
            n112 = Unbundle By Name(w321) -> ("Self Reference"=w319:refnum<class "JKI.Robot.SMO.APITesterUI.lvclass">)
            n113 = Bundle By Name(cluster=w321, "Self Reference"=w319) -> (w320:T4)
            n114 = call <vilib>:"Add State(s) to Queue__jki_lib_state_machine.vi"("State(s) in (\"\")"=w325) -> ("States Out"=w324:string)  [unwired: 14 in]
          }
          frame "Action: Notify UI Closed" {
            # "Notify that the UI has been closed"
            n115 = Unbundle By Name(w328) -> ("Self Reference"=w329:refnum<class "JKI.Robot.SMO.APITesterUI.lvclass">)
            n116 = call <vilib>:"Hide.vi"("error in (no error)"=w327, "SMO.UI"=w329) -> ("error out"=w326:errorcluster)  [unwired: 8 in, 1 out]
            n117 = call <vilib>:"Add State(s) to Queue__jki_lib_state_machine.vi"("State(s) in (\"\")"=w332) -> ("States Out"=w331:string)  [unwired: 14 in]
          }
        }
      }
    }
    frame Error {
    }
  }
  n118 = call-parent "Process.vi"("error in (no error)"=w8, "SMO.UI"=w7) -> ("error out"=w5:errorcluster, "SMO.UI out"=→"JKI.Robot.SMO.TestUI out":refnum<class "JKI.Robot.SMO.APITesterUI.lvclass">)  [unwired: 8 in]
  n119 = Merge Errors(w5, w4) -> (→"error out":errorcluster)
